vi "WK6425_CommandsGlobal.vi"() -> ()   [LabVIEW 2019, in "WK6425.lvclass"]
uses:
  WK6425.lvclass
panel:
  in  "WayneKerr 6425 GPIB Setup":T1={"Instrument name"="WayneKerr 6425", "Command \"Initialise LCR\""="%s;FREQ%d;LEV%1.2fV;AUT;NORS;C;TRG", "Command \"OC Trim\""="TOC", "Command \"LCR Readout\""="TRG"}
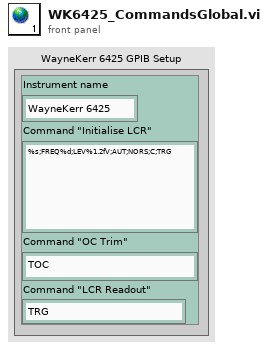
[diagram p1: front panel]
types:
  T1 = cluster{"Instrument name":string, "Command \"Initialise LCR\"":string, "Command \"OC Trim\"":string, "Command \"LCR Readout\"":string}
diagram:
